vi "Autonomous Independent.vi"() -> ()   [LabVIEW 2019]
doc: "This VI is called when autonomous begins, and will automatically be terminated when autonomous ends. You can carry out timed or sensor driven robot movement independently without needing to return to the caller."
uses:
  <vilib>/Rock Robotics/WPI/Utilities/WPI_GetSetVariantRefNum.vi
  <vilib>/Rock Robotics/Network Tables/NT Read String.vi
  <vilib>/Rock Robotics/WPI/RobotDrive/WPI_RobotDriveArcadeDrive_Standard(NoSaturation).vi
panel:
  out "Current Movement, for debugging":T1 {"Y Joystick Value" scale=1.0..-1.0; "X Joystick Value" scale=-1.0..1.0}
  in  "Array of robot movements":T2(array[cluster])=[{"X Joystick Value"=0.39393939393939403, "Y Joystick Value"=0.0, "Delay (sec)"=1.0, "Movement Name"="turn"}, {"X Joystick Value"=-0.3737373737373737, "Y Joystick Value"=0.0, "Delay (sec)"=1.0, "Movement Name"="turn back"}] {"Y Joystick Value" scale=1.0..-1.0; "X Joystick Value" scale=-1.0..1.0}
  # "Be sure to right-click and choose Data Operations>>Make Current Value default if you want to save the array values with the VI"
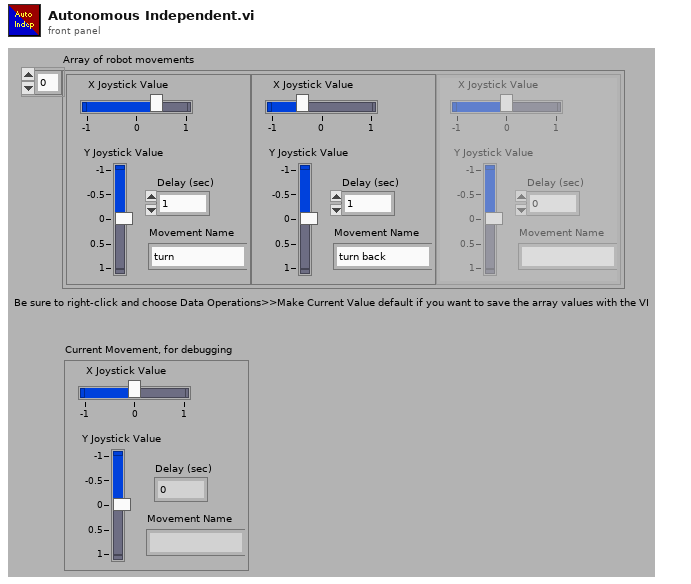
[diagram p1: front panel]
types:
  T1 = cluster{"X Joystick Value":dbl, "Y Joystick Value":dbl, "Delay (sec)":dbl, "Movement Name":string}
  T2 = cluster{"X Joystick Value":dbl, "Y Joystick Value":dbl, "Delay (sec)":dbl, "Movement Name":string}[]
  T3 = typedef "WPI_JoystickDevRef.ctl" = cluster{"Device":T4}
  T4 = typedef "WPI_JoystickDeviceEnum.ctl" = enum16{"USB 0", "USB 1", "USB 2", "USB 3", "USB 4", "USB 5"}
  T5 = typedef "WPI_RobotDriveDevRef.ctl" = cluster{"DevStatus":errorcluster, "Motors[]":T6[], "Square Inputs":bool, "Max Output":dbl}
  T6 = typedef "WPI_MotorControlDeviceRef.ctl" = cluster{"DeviceStatus":errorcluster, "Type":T7, "PWM":cluster{"PWM Channel":T8, "DeadBand":T9}, "CAN":cluster{"Device Number":u8, "SetOutput VI Ref":variant, "GetOutput VI Ref":variant, "Enable VI Ref":variant, "Disable VI Ref":variant, "Data":variant}, "Invert":bool, "DIO PWM":cluster{"PWM \"Enable\" Channel":T8, "DIOChannel":T10, "PWM Rate":dbl}}
  T7 = typedef "WPI_MotorControlType.ctl" = enum16{"PWM", "CAN", "DIO PWM"}
  T8 = typedef "FPGA_DIOPWMChannel.ctl" = enum8{"PWM 0", "PWM 1", "PWM 2", "PWM 3", "PWM 4", "PWM 5", "PWM 6", "PWM 7", "PWM 8", "PWM 9", "PWM MXP 0", "PWM MXP 1", "PWM MXP 2", "PWM MXP 3", "PWM MXP 4", "PWM MXP 5", "PWM MXP 6", "PWM MXP 7", "PWM MXP 8", "PWM MXP 9", "Invalid"}
  T9 = typedef "WPI_PWMDeadband.ctl" = cluster{"Name":string, "maxPositivePwm":i32, "minPositivePwm":i32, "centerPwm":i32, "maxNegativePwm":i32, "minNegativePwm":i32, "angularRange":u16}
  T10 = typedef "FPGA_DIOChannel.ctl" = enum8{"DIO 0", "DIO 1", "DIO 2", "DIO 3", "DIO 4", "DIO 5", "DIO 6", "DIO 7", "DIO 8", "DIO 9", "DIO MXP 0", "DIO MXP 1", "DIO MXP 2", "DIO MXP 3", "DIO MXP 4", "DIO MXP 5", "DIO MXP 6", "DIO MXP 7", "DIO MXP 8", "DIO MXP 9", "DIO MXP 10", "DIO MXP 11", "DIO MXP 12", "DIO MXP 13", "DIO MXP 14", "DIO MXP 15", "SPI Port CS1", "SPI Port CS2", "SPI Port CS3", "SPI Port MISO", "SPI Port MOSI", "Invalid"}
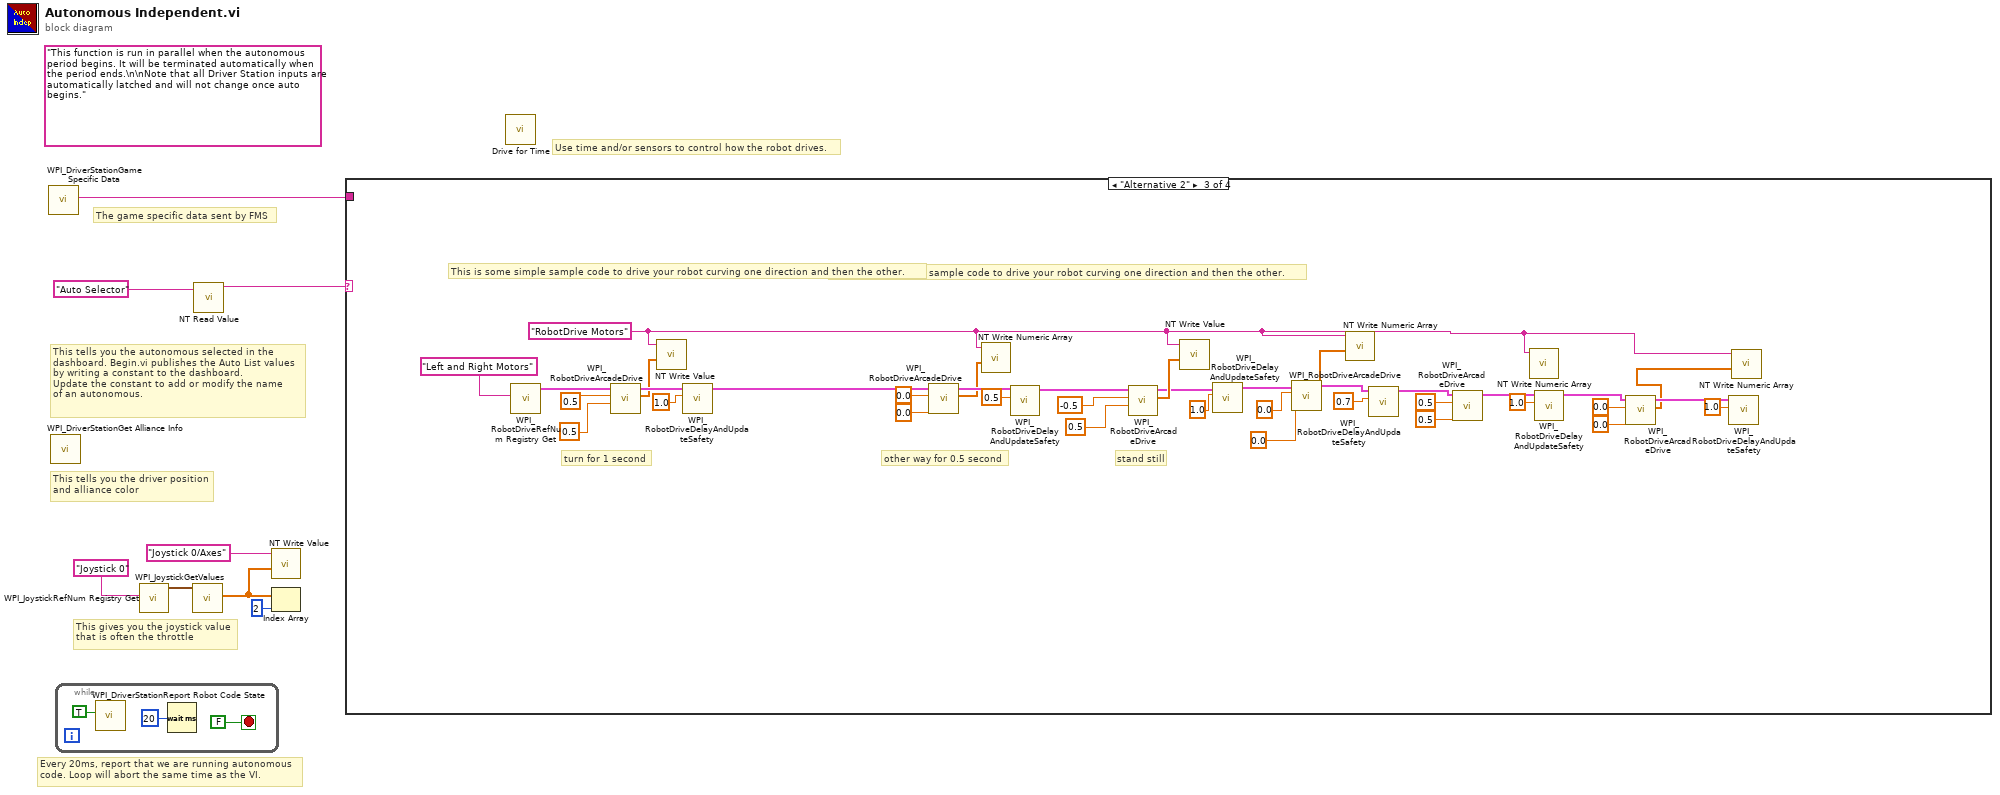
[diagram p0: block diagram]
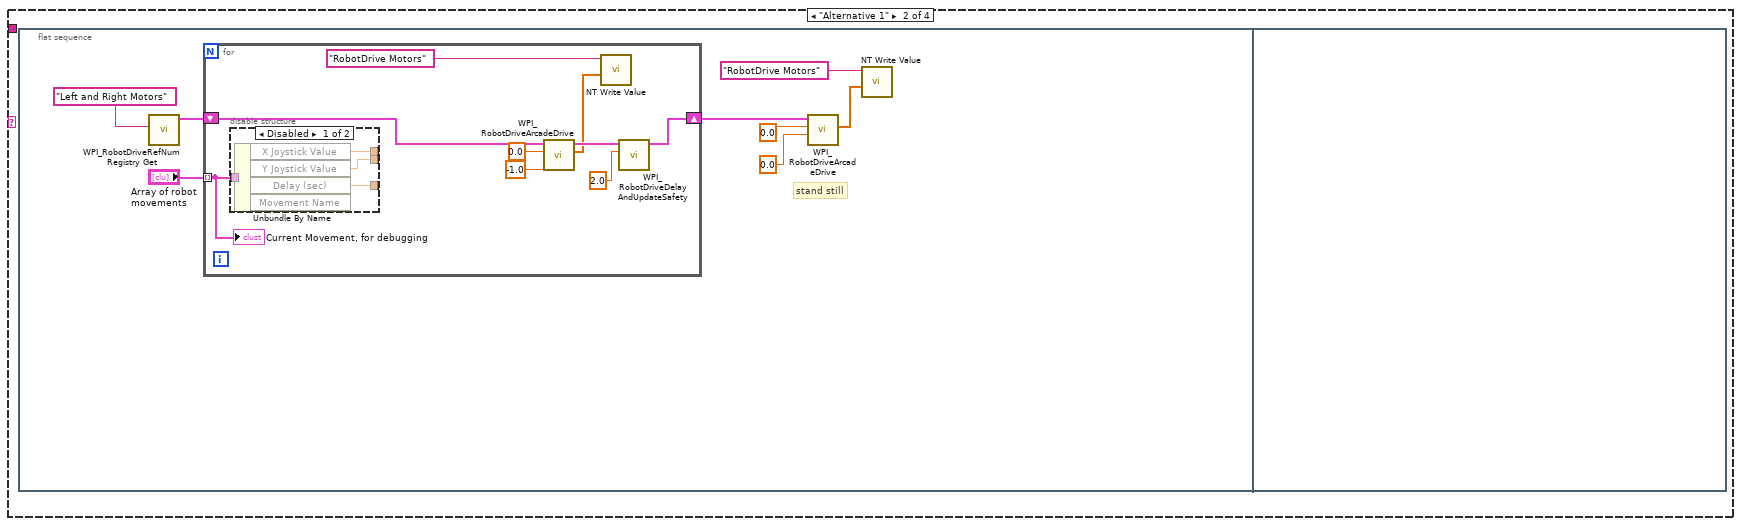
[diagram p3: hidden frame]
diagram:
  (unwired) "This function is run in parallel when the autonomous period begins. It will be terminated automatically when the period ends.\n\nNote that all Driver Station inputs are automatically latched and will not change once auto begins."
  # "The game specific data sent by FMS"
  # "This tells you the autonomous selected in the \ndashboard. Begin.vi publishes the Auto List values\nby writing a constant to the dashboard.\nUpdate the constant to add or modify the name\nof an autonomous."
  # "Every 20ms, report that we are running autonomous\ncode. Loop will abort the same time as the VI."
  # "This gives you the joystick value\nthat is often the throttle"
  # "Use time and/or sensors to control how the robot drives."
  # "This tells you the driver position\nand alliance color"
  n1 = call <vilib>:"WPI_DriverStationGame Specific Data.vi"() -> ("Game Specific Data"=w1:string)  [unwired: 11 in]
  n2 = call <vilib>:"WPI_DriverStationGet Alliance Info.vi"() -> ()  [unwired: 12 out]
  n3 = while {
    stop <- FALSE stop-if-true
    n4 = call <vilib>:"WPI_DriverStationReport Robot Code State.vi"("Autonomous"=TRUE) -> ()  [unwired: 10 in, 1 out]
    n5 = Wait (ms)(milliseconds to wait=u32 20) -> ()  [unwired: 1 out]
  }
  n6 = call <vilib>:"WPI_JoystickRefNum Registry Get.vi"("refnum name"="Joystick 0") -> ("JoystickDevRef"=w7:T3)  [unwired: 1 in, 9 out]
  n7 = call <vilib>:"WPI_JoystickGetValues.vi"("JoystickDevRef"=w7) -> ("Axes"=w3:dbl[])  [unwired: 6 in, 4 out]
  n8 = call-poly <vilib>:"NT Read Value.vi"("Name"="Auto Selector") -> ("String"=w4:string)  [unwired: 9 in, 1 out]
  n9 = call-poly <vilib>:"NT Write Value.vi"("Numeric Array"=w3, "Name"="Joystick 0/Axes") -> ()  [unwired: 9 in, 1 out]
  n10 = Index Array(array=w3, index=2) -> ()  [unwired: 1 out]
  n11 = case shown="\"Alternative 2\"" w4 {
    tunnel: w1 -> [_ _ _ _]
    frame Default {
      # "You can put your main auto here, or you can right-click on the case and make any\nother frame be the default case."
      # "This is the frame that will execute if no selection is made, or if it is not recognized"
      n12 = flat-sequence {
        frame #0 {
        }
        frame #1 {
        }
      }
    }
    frame "Alternative 1" {
      n13 = flat-sequence {
        frame #0 {
          # "stand still"
          n14 = call <vilib>:"WPI_RobotDriveRefNum Registry Get.vi"("refnum name"="Left and Right Motors") -> ("RobotDriveDevRef"=w18:T5)  [unwired: 1 in, 9 out]
          n15 = for {
            shift-right: [w26] -> w13
            shift-left: w18 -> [w27]
            tunnel: "Array of robot movements" -> [w24] mode=indexing
            n16 = disable-structure shown="Disabled" {
              disable-tunnel: [w32 _] -> _
              disable-tunnel: w24 -> [w31 _]
              disable-tunnel: [w30 _] -> _
              disable-tunnel: [w29 _] -> _
              frame Disabled {
                n17 = Unbundle By Name(w31) -> ("X Joystick Value"=w30:dbl, "Y Joystick Value"=w29:dbl, "Delay (sec)"=w32:dbl)  [unwired: 1 out]
              }
              frame Enabled {
              }
            }
            n18 = call-poly <vilib>:"WPI_RobotDriveArcadeDrive.vi"("Y axis value"=-1.0, "X axis value"=0.0, "RobotDriveDevRef"=w27) -> ("Motor Values"=w22:dbl[], "RobotDriveDevRef"=w28:T5)  [unwired: 1 in, 6 out]
            n19 = call-poly <vilib>:"NT Write Value.vi"("Numeric Array"=w22, "Name"="RobotDrive Motors") -> ()  [unwired: 9 in, 1 out]
            n20 = call <vilib>:"WPI_RobotDriveDelayAndUpdateSafety.vi"("Delay (s)"=2.0, "RobotDriveDevRef"=w28) -> ("RobotDriveDevRef 2"=w26:T5)  [unwired: 8 in, 1 out]
            "Current Movement, for debugging" <- w24
          }
          n21 = call-poly <vilib>:"WPI_RobotDriveArcadeDrive.vi"("Y axis value"=0.0 ("X axis value"), "X axis value"=0.0, "RobotDriveDevRef"=w13) -> ("Motor Values"=w16:dbl[])  [unwired: 1 in, 7 out]
          n22 = call-poly <vilib>:"NT Write Value.vi"("Numeric Array"=w16, "Name"="RobotDrive Motors") -> ()  [unwired: 9 in, 1 out]
        }
        frame #1 {
        }
      }
    }
    frame "Alternative 2" {
      w34 = "RobotDrive Motors" ("Name")
      # "This is some simple sample code to drive your robot curving one direction and then the other."
      # "This is some simple sample code to drive your robot curving one direction and then the other."
      # "stand still"
      # "other way for 0.5 second"
      # "turn for 1 second"
      n23 = call <vilib>:"WPI_RobotDriveRefNum Registry Get.vi"("refnum name"="Left and Right Motors") -> ("RobotDriveDevRef"=w69:T5)  [unwired: 1 in, 9 out]
      n24 = call-poly <vilib>:"WPI_RobotDriveArcadeDrive.vi"("Y axis value"=0.5 ("X axis value"), "X axis value"=0.5, "RobotDriveDevRef"=w69) -> ("Motor Values"=w58:dbl[], "RobotDriveDevRef"=w63:T5)  [unwired: 1 in, 6 out]
      n25 = call-poly <vilib>:"NT Write Value.vi"("Numeric Array"=w58, "Name"=w34) -> ()  [unwired: 9 in, 1 out]
      n26 = call <vilib>:"WPI_RobotDriveDelayAndUpdateSafety.vi"("Delay (s)"=1.0, "RobotDriveDevRef"=w63) -> ("RobotDriveDevRef 2"=w64:T5)  [unwired: 8 in, 1 out]
      n27 = call-poly <vilib>:"WPI_RobotDriveArcadeDrive.vi"("Y axis value"=0.0, "X axis value"=0.0, "RobotDriveDevRef"=w64) -> ("Motor Values"=w57:dbl[], "RobotDriveDevRef"=w65:T5)  [unwired: 1 in, 6 out]
      n28 = call <vilib>:"NT Write Numeric Array.vi"("Numeric Array"=w57, "Name"=w34) -> ()  [unwired: 9 in, 1 out]
      n29 = call <vilib>:"WPI_RobotDriveDelayAndUpdateSafety.vi"("Delay (s)"=0.5, "RobotDriveDevRef"=w65) -> ("RobotDriveDevRef 2"=w66:T5)  [unwired: 8 in, 1 out]
      n30 = call-poly <vilib>:"WPI_RobotDriveArcadeDrive.vi"("Y axis value"=0.5 ("X axis value"), "X axis value"=-0.5, "RobotDriveDevRef"=w66) -> ("Motor Values"=w53:dbl[], "RobotDriveDevRef"=w52:T5)  [unwired: 1 in, 6 out]
      n31 = call-poly <vilib>:"NT Write Value.vi"("Numeric Array"=w53, "Name"=w34) -> ()  [unwired: 9 in, 1 out]
      n32 = call <vilib>:"WPI_RobotDriveDelayAndUpdateSafety.vi"("Delay (s)"=1.0, "RobotDriveDevRef"=w52) -> ("RobotDriveDevRef 2"=w50:T5)  [unwired: 8 in, 1 out]
      n33 = call-poly <vilib>:"WPI_RobotDriveArcadeDrive.vi"("Y axis value"=0.0, "X axis value"=0.0, "RobotDriveDevRef"=w50) -> ("Motor Values"=w49:dbl[], "RobotDriveDevRef"=w45:T5)  [unwired: 1 in, 6 out]
      n34 = call <vilib>:"NT Write Numeric Array.vi"("Numeric Array"=w49, "Name"=w34) -> ()  [unwired: 9 in, 1 out]
      n35 = call <vilib>:"WPI_RobotDriveDelayAndUpdateSafety.vi"("Delay (s)"=0.7, "RobotDriveDevRef"=w45) -> ("RobotDriveDevRef 2"=w44:T5)  [unwired: 8 in, 1 out]
      n36 = call-poly <vilib>:"WPI_RobotDriveArcadeDrive.vi"("Y axis value"=0.5, "X axis value"=0.5, "RobotDriveDevRef"=w44) -> ("RobotDriveDevRef"=w43:T5)  [unwired: 1 in, 7 out]
      n37 = call <vilib>:"NT Write Numeric Array.vi"("Name"=w34) -> ()  [unwired: 10 in, 1 out]
      n38 = call <vilib>:"WPI_RobotDriveDelayAndUpdateSafety.vi"("Delay (s)"=1.0, "RobotDriveDevRef"=w43) -> ("RobotDriveDevRef 2"=w39:T5)  [unwired: 8 in, 1 out]
      n39 = call-poly <vilib>:"WPI_RobotDriveArcadeDrive.vi"("Y axis value"=0.0, "X axis value"=0.0, "RobotDriveDevRef"=w39) -> ("Motor Values"=w33:dbl[], "RobotDriveDevRef"=w38:T5)  [unwired: 1 in, 6 out]
      n40 = call <vilib>:"WPI_RobotDriveDelayAndUpdateSafety.vi"("Delay (s)"=1.0, "RobotDriveDevRef"=w38) -> ()  [unwired: 8 in, 2 out]
      n41 = call <vilib>:"NT Write Numeric Array.vi"("Numeric Array"=w33, "Name"=w34) -> ()  [unwired: 9 in, 1 out]
    }
    frame "Your Turn" {
    }
  }
  n42 = call "Drive for Time.vi"() -> ()  [unwired: 11 in, 1 out]
